vi "1-at-a-time(SubVI).vi"(8 "error in (no error)":errorcluster, 9 "Wait Between Characters(ms)":u32=4, 10 "write buffer":string, 11 "VISA resource name":refnum<visa-resource-name>) -> (0 "error out":errorcluster, 2 "Return Count":u32, 3 "VISA resource name out":refnum<visa-resource-name>)   [LabVIEW 2017]
doc: "For Instruments that require characters to be written one at a time. It breaks down the string into individual bytes and transfers one at a time."
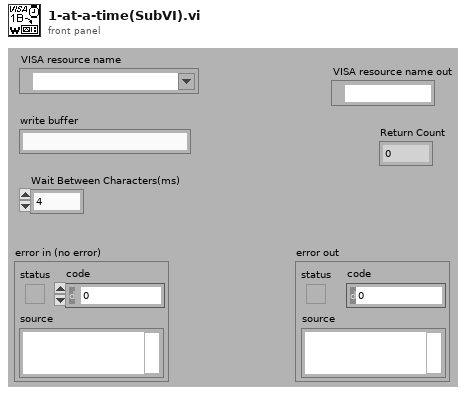
[diagram p1: front panel]
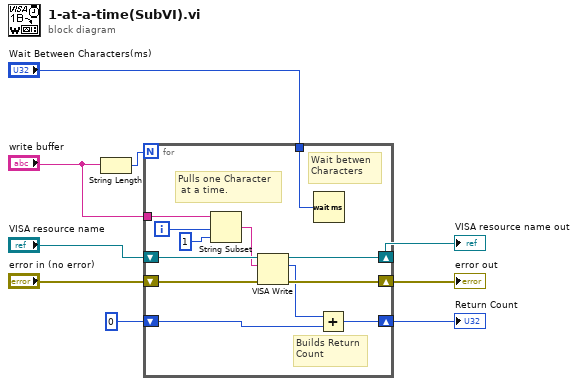
[diagram p0: block diagram]
diagram:
  n1 = String Length(string="write buffer") -> (length=w2:i32)
  n2 = for {
    N: w2 -> [_]
    shift-right: [w18] -> w6
    shift-left: "VISA resource name" -> [w19]
    shift-right: [w20] -> w8
    shift-left: "error in (no error)" -> [w21]
    shift-right: [w16] -> w3
    shift-left: u32 0 -> [w15]
    tunnel: "Wait Between Characters(ms)" -> [w14]
    tunnel: "write buffer" -> [w11]
    i -> [w13]
    # "Wait betwen \nCharacters"
    # "Builds Return\nCount"
    # "Pulls one Character\n at a time."
    n3 = String Subset(string=w11, offset (0)=w13, length (rest)=1 ("length (rest)")) -> (substring=w10:string)
    n4 = VISA Write(VISA resource name=w19, write buffer=w10, error in (no error)=w21) -> (VISA resource name out=w18:refnum<visa-resource-name>, return count=w17:u32, error out=w20:errorcluster)
    n5 = Wait (ms)(milliseconds to wait=w14) -> ()  [unwired: 1 out]
    n6 = Add(x=w17, y=w15) -> (x+y=w16:u32)
  }
  "error out" <- w8
  "VISA resource name out" <- w6
  "Return Count" <- w3
